vi "predict_score.vi"(10 "feature":dbl[](array[numeric])) -> (2 "predict":dbl format="%.2f")   [LabVIEW 2018]
uses:
  <vilib>/Analysis/NI_AALBase.lvlib
  <vilib>/Analysis/baseanly.llb/Real Dot Product.vi
  <vilib>/Analysis/baseanly.llb/Vector x A.vi
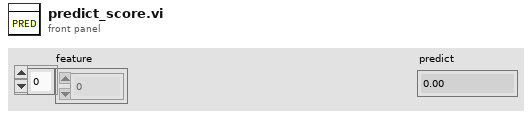
[diagram p1: front panel]
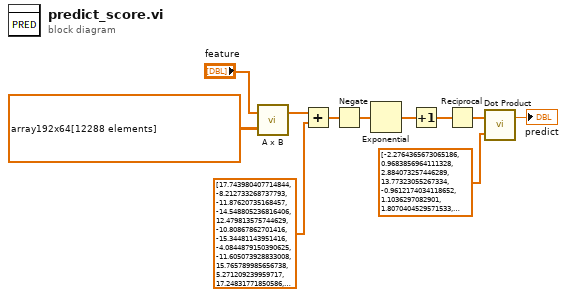
[diagram p0: block diagram]
diagram:
  n1 = call-poly <vilib>:"A x B.vi"("Matrix A"=dbl[][] array192x64[12288 elements] ("transposed array"), "Vector V'"="feature") -> ("V' x A"=w8:dbl[])  [unwired: 1 out]
  n2 = Add(x=w8, y=dbl[] [17.743980407714844, -8.212733268737793, -11.87620735168457, -14.548805236816406, 12.479813575744629, -10.80867862701416, -15.34481143951416, -4.0844879150390625, -11.605073928833008, 15.765789985656738, 5.271209239959717, 17.24831771850586, -13.033778190612793, -11.343328475952148, 12.904179573059082, -4.485091209411621, 18.403371810913086, 22.437788009643555, 12.106035232543945, -4.996275901794434, -1.0242927074432373, -13.932183265686035, 15.209809303283691, -10.585172653198242, -3.0788233280181885, 7.993998050689697, 3.22343111038208, 12.245124816894531, -11.954809188842773, 10.889013290405273, 0.24468061327934265, 8.666336059570312, -19.683595657348633, -19.2744197845459, -14.961505889892578, -10.869546890258789, 12.225735664367676, -23.41131591796875, -0.9478909373283386, 16.29218292236328, 6.5120062828063965, -10.294530868530273, 6.243919849395752, 17.50108528137207, 4.4055562019348145, -14.003582954406738, 16.81816291809082, -14.93195915222168, -11.365662574768066, -8.830365180969238, -4.254379749298096, 16.312271118164062, 14.19776725769043, -11.391602516174316, 6.946492671966553, 11.063065528869629, 14.21729564666748, -18.89331817626953, -3.7810065746307373, 10.302671432495117, -3.052011728286743, 17.959381103515625, -14.757219314575195, 5.421353816986084] ("subarray")) -> (x+y=w6:dbl[])
  n3 = Negate(x=w6) -> (-x=w10:dbl[])
  n4 = Exponential(1:w10) -> (0:w9:dbl[])
  n5 = Increment(x=w9) -> (x+1=w5:dbl[])
  n6 = Reciprocal(x=w5) -> (1/x=w4:dbl[])
  n7 = call-poly <vilib>:"Dot Product.vi"("Y Vector"=dbl[] [-2.2764365673065186, 0.9683856964111328, 2.884073257446289, 13.77323055267334, -0.9612174034118652, 1.1036297082901, 1.8070404529571533, 1.816266417503357, 1.7829430103302002, -1.2620164155960083, -1.3441156148910522, -1.8231568336486816, 1.331135630607605, 1.2457172870635986, -0.9199069738388062, 1.3182203769683838, -1.8270713090896606, -1.4839565753936768, -2.119565725326538, 3.288271903991699, -0.208245649933815, 1.474808931350708, -1.6956777572631836, 2.2918083667755127, 1.6890760660171509, -2.341543436050415, -2.2623581886291504, -1.3775190114974976, 1.3595422506332397, -0.7426940202713013, -1.5588895082473755, -2.464414596557617, 10.103519439697266, 1.5024877786636353, 2.1463301181793213, 1.9694830179214478, -3.0613198280334473, 5.444678783416748, -1.4442726373672485, -2.218681812286377, -0.9395902156829834, 1.1766349077224731, -2.251075029373169, -1.0036507844924927, -0.5509436130523682, 1.3056422472000122, -1.003251552581787, 2.1590261459350586, 1.7256617546081543, 2.080587863922119, -0.759282112121582, -1.6064882278442383, -1.9997947216033936, 2.8963232040405273, -0.8096559047698975, -1.034389615058899, -1.736072301864624, 1.9859275817871094, 1.6924716234207153, -0.9035972356796265, -0.7430725693702698, -1.0748728513717651, 1.692287802696228, -5.6733622550964355] ("subarray 2"), "X Vector"=w4) -> ("X * Y"=→"predict":dbl)  [unwired: 1 out]
